vi "Echo_Begin.vi"(10 "Read":bool, 11 "Files":path[](array[path])) -> ()   [LabVIEW 2012]
uses:
  Echo_Global_Data.vi
  <vilib>/Utility/file.llb/Read From Spreadsheet File (DBL).vi
panel:
  # "This VI is contained within Echo Periodic Tasks,\nand Echo Disabled\n\nIt takes an input array of file paths, and uses\nthem to generate a 3D array that represents\nthe autonomous routine (Echo Combined Data)"
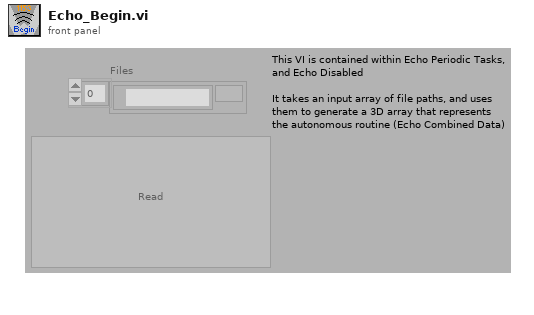
[diagram p1: front panel]
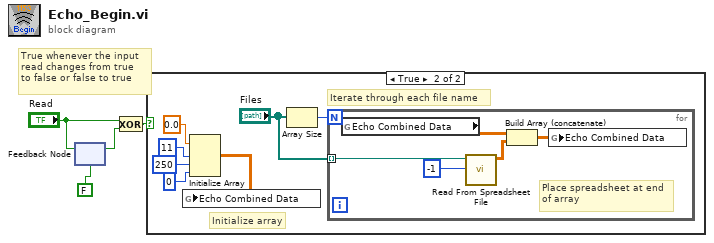
[diagram p0: block diagram]
diagram:
  # "True whenever the input\nread changes from true \nto false or false to true"
  n1 = feedback-in #1("Read") -> ()
  n2 = feedback #1(FALSE ("Read")) -> (w2:bool)
  n3 = Exclusive Or(1:w2, 2:"Read") -> (0:w4:bool)
  n4 = case shown="True" w4 {
    frame False {
    }
    frame True {
      # "Iterate through each file name"
      # "Initialize array"
      n5 = Initialize Array(0.0 ("element"), 11 ("dimension size"), 250 ("dimension size"), 0 ("dimension size")) -> (w6:dbl[][][])
      n6 = global write "Echo_Global_Data.vi" "Echo Combined Data"(w6) -> ()
      n7 = Array Size(array="Files") -> (size(s)=w11:i32)
      n8 = for {
        N: w11 -> [_]
        tunnel: "Files" -> [w13] mode=indexing
        # "Place spreadsheet at end\nof array"
        n9 = global read "Echo_Global_Data.vi" "Echo Combined Data"() -> (w15:dbl[][][])
        n10 = call-poly <vilib>:"Read From Spreadsheet File.vi"("number of rows (all:-1)"=-1, "file path (dialog if empty)"=w13) -> ("all rows"=w14:dbl[][])  [unwired: 2 in, 7 out]
        n11 = Build Array (concatenate)(w15, w14) -> (w12:dbl[][][])
        n12 = global write "Echo_Global_Data.vi" "Echo Combined Data"(w12) -> ()
      }
    }
  }
